vi "To String.vi"(8 "error in (no error)":errorcluster, 11 "JSON Boolean in":refnum<class "JSON Boolean.lvclass">) -> (0 "error out":errorcluster, 3 "String":string)   [LabVIEW 2017, in "LVJSON.lvlib" / "JSON Boolean.lvclass"]
uses:
  JSON Boolean.lvclass
  JSON Boolean.lvclass/JSON Boolean.ctl
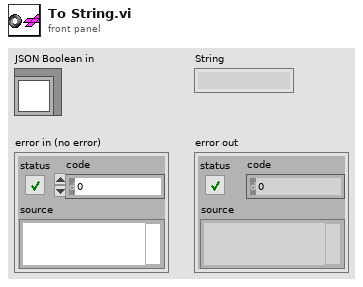
[diagram p1: front panel]
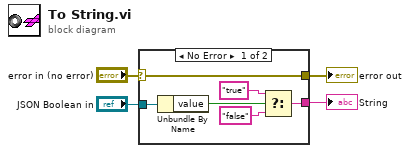
[diagram p0: block diagram]
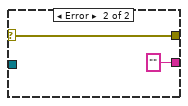
[diagram p2: hidden frame]
diagram:
  n1 = case shown="No Error" "error in (no error)" {
    selector: "error in (no error)" -> [w5 w11]
    tunnel: "JSON Boolean in" -> [w10 _]
    tunnel: [w6 "" ("f")] -> w3
    tunnel: [w5 w11] -> w1
    frame No Error {
      n2 = Unbundle By Name(w10) -> ("value"=w9:bool)
      n3 = Select(t="true" ("String"), s=w9, f="false") -> (s? t:f=w6:string)
    }
    frame Error {
    }
  }
  "String" <- w3
  "error out" <- w1
